vi "Write user settings.vi"(8 "error in (no error)":errorcluster, 10 "user settings":variant, 11 "DSFPluginSettings in":refnum<class "DSFPluginSettings.lvclass">) -> (0 "error out":errorcluster, 3 "DSFPluginSettings out":refnum<class "DSFPluginSettings.lvclass">)   [LabVIEW 2017, in "DSFPluginSettings.lvclass"]
uses:
  DSFPluginSettings.lvclass
  DSFPluginSettings.lvclass/DSFPluginSettings.ctl
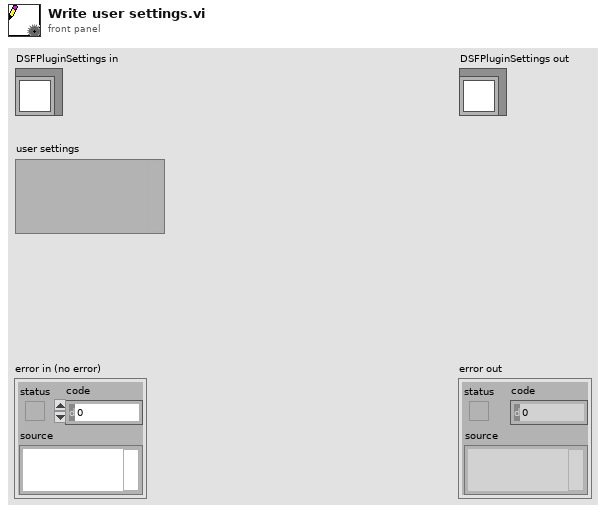
[diagram p1: front panel]
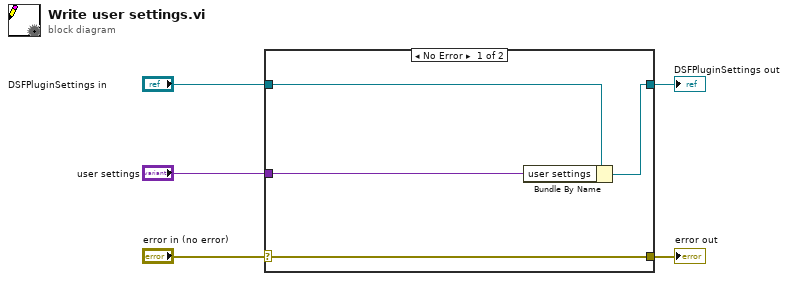
[diagram p0: block diagram]
diagram:
  n1 = case shown="No Error" "error in (no error)" {
    selector: "error in (no error)" -> [w9 w10]
    tunnel: [w9 w10] -> w4
    tunnel: [w7 w11] -> w2
    tunnel: "DSFPluginSettings in" -> [w8 w11]
    tunnel: "user settings" -> [w6 _]
    frame No Error {
      n2 = Bundle By Name(cluster=w8, "user settings"=w6) -> (w7:refnum<class "DSFPluginSettings.lvclass">)
    }
    frame Error {
    }
  }
  "error out" <- w4
  "DSFPluginSettings out" <- w2
